vi "type_20_string_one_segment.vi"() -> ()   [LabVIEW 2010]
panel:
  out "error out":errorcluster
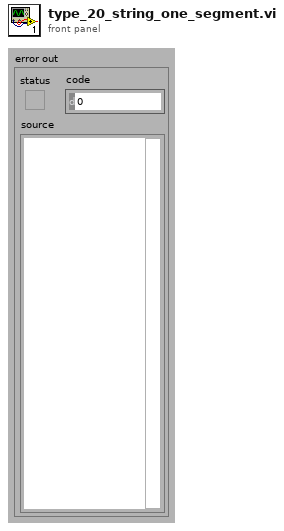
[diagram p1: front panel]
types:
  T1 = enum16{"open", "open or create", "create or replace", "create", "open (read-only)"}
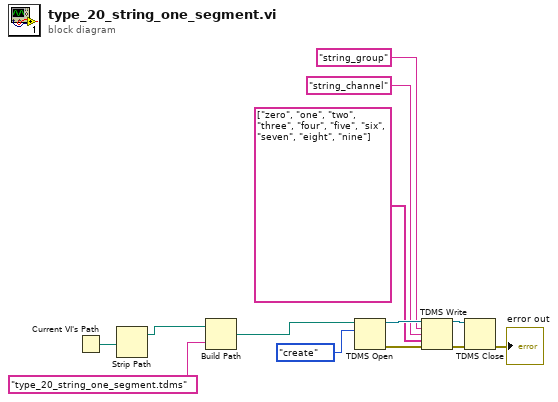
[diagram p0: block diagram]
diagram:
  n1 = Current VI's Path() -> (path=w4:path)
  n2 = Strip Path(path=w4) -> (stripped path=w3:path)  [unwired: 1 out]
  n3 = Build Path(base path=w3, name or relative path="type_20_string_one_segment.tdms") -> (appended path=w1:path)
  n4 = TDMS Open(10:T1."create" ("operation (0:open)"), 11:w1) -> (0:w13:errorcluster, 3:w12:refnum<k34>)  [unwired: 4 in]
  n5 = TDMS Write(0:w12, 5:"string_group" ("group name in (Untitled)"), 7:"string_channel" ("channel name(s) in (Untitled)"), 9:string[] ["zero", "one", "two", "three", "four", "five", "six", "seven", "eight", "nine"] ("channel name(s) in (Untitled)"), 11:w13) -> (4:w7:refnum<k34>, 15:w6:errorcluster)  [unwired: 1 in, 2 out]
  n6 = TDMS Close(8:w6, 11:w7) -> (0:→"error out":errorcluster)  [unwired: 1 out]
